vi "test_Checksum U8 - Add Protection.vi"(8 "error in (no error)":errorcluster) -> (0 "error out":errorcluster)   [LabVIEW 2019, in "Protections Unit Tests.lvclass"]
uses:
  Protections Unit Tests.lvclass
  Checksum U8/Checksum U8.lvclass
  <vilib>/addons/_JKI Toolkits/VI Tester/TestCase.llb/TestCase.lvclass
  C:/Program Files (x86)/National Instruments/LabVIEW 2019/vi.lib/addons/_JKI Toolkits/VI Tester/TestCase.llb/TestCase.lvclass
panel:
  out "Checksum U8 out":refnum<class "Checksum U8.lvclass">
  in  "Checksum U8 in":refnum<class "Checksum U8.lvclass">
  out "TestCase out":refnum<class "Protections Unit Tests.lvclass">
  in  "TestCase in":refnum<class "Protections Unit Tests.lvclass">
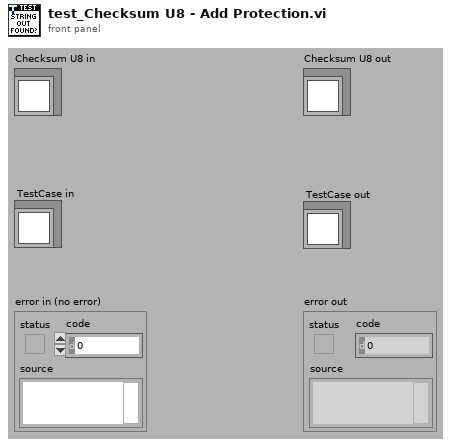
[diagram p1: front panel]
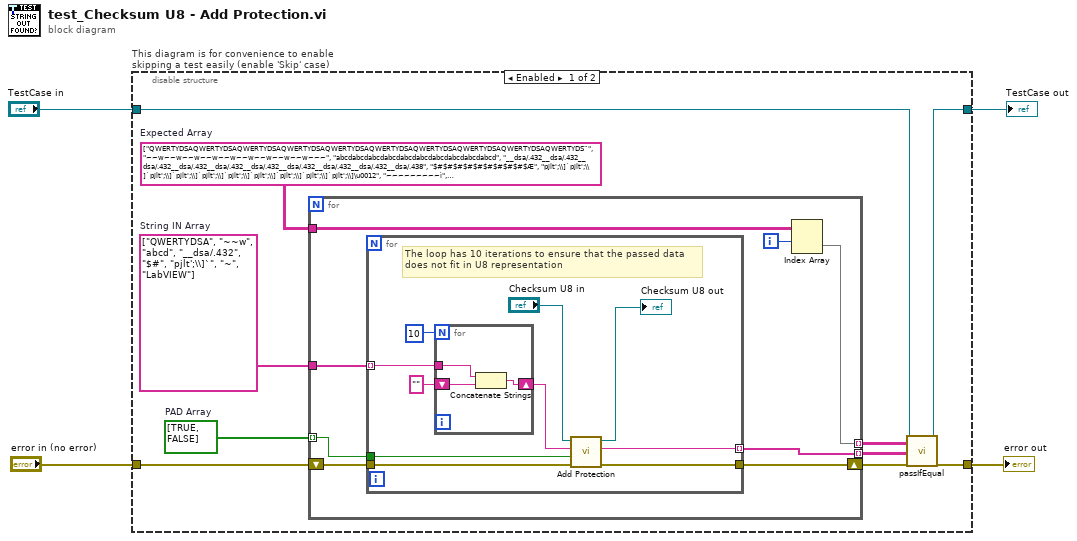
[diagram p0: block diagram]
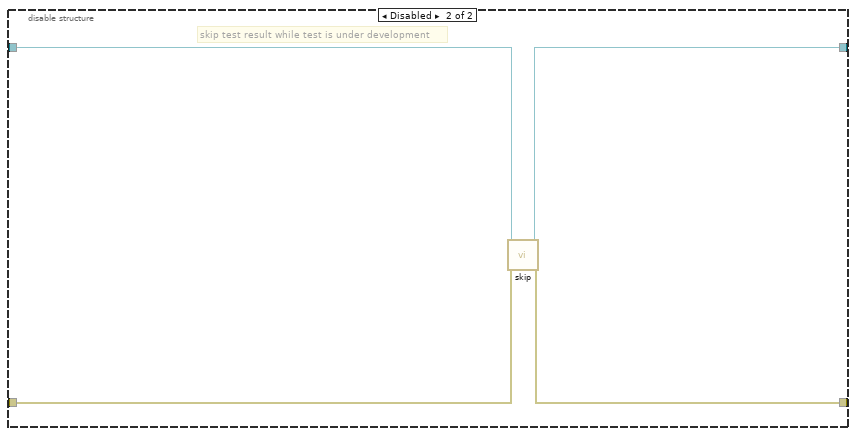
[diagram p2: hidden frame]
diagram:
  n1 = disable-structure "This diagram is for convenience to enable skipping a test easily (enable 'Skip' case)" shown="Enabled" {
    disable-tunnel: "TestCase in" -> [w12 w39]
    disable-tunnel: [w13 w37] -> w1
    disable-tunnel: [w14 w38] -> w3
    disable-tunnel: "error in (no error)" -> [w11 w36]
    frame Enabled {
      w5 = string[][] [["QWERTYDSAQWERTYDSAQWERTYDSAQWERTYDSAQWERTYDSAQWERTYDSAQWERTYDSAQWERTYDSAQWERTYDSAQWERTYDS¨", "~~w~~w~~w~~w~~w~~w~~w~~w~~w~~~", "abcdabcdabcdabcdabcdabcdabcdabcdabcdabcd", "__dsa/.432__dsa/.432__dsa/.432__dsa/.432__dsa/.432__dsa/.432__dsa/.432__dsa/.432__dsa/.432__dsa/.438", "$#$#$#$#$#$#$#$#$#$Æ", "pjlt';\\]`pjlt';\\]`pjlt';\\]`pjlt';\\]`pjlt';\\]`pjlt';\\]`pjlt';\\]`pjlt';\\]`pjlt';\\]`pjlt';\\]\u0012", "~~~~~~~~~ì", "LabVIEWLabVIEWLabVIEWLabVIEWLabVIEWLabVIEWLabVIEWLabVIEWLabVIEWLabVIEä"], ["QWERTYDSAQWERTYDSAQWERTYDSAQWERTYDSAQWERTYDSAQWERTYDSAQWERTYDSAQWERTYDSAQWERTYDSAQWERTYDSA¨", "~~w~~w~~w~~w~~w~~w~~w~~w~~w~~w~", "abcdabcdabcdabcdabcdabcdabcdabcdabcdabcdd", "__dsa/.432__dsa/.432__dsa/.432__dsa/.432__dsa/.432__dsa/.432__dsa/.432__dsa/.432__dsa/.432__dsa/.4328", "$#$#$#$#$#$#$#$#$#$#Æ", "pjlt';\\]`pjlt';\\]`pjlt';\\]`pjlt';\\]`pjlt';\\]`pjlt';\\]`pjlt';\\]`pjlt';\\]`pjlt';\\]`pjlt';\\]`\u0012", "~~~~~~~~~~ì", "LabVIEWLabVIEWLabVIEWLabVIEWLabVIEWLabVIEWLabVIEWLabVIEWLabVIEWLabVIEWä"]]  # Expected Array
      w7 = string[] ["QWERTYDSA", "~~w", "abcd", "__dsa/.432", "$#", "pjlt';\\]`", "~", "LabVIEW"]  # String IN Array
      w8 = bool[] [TRUE, FALSE]  # PAD Array
      n2 = for {
        tunnel: [w21] -> w10 mode=indexing
        shift-right: [w20] -> w9
        shift-left: w11 -> [w22]
        tunnel: w8 -> [w19] mode=indexing
        tunnel: w7 -> [w18]
        tunnel: w5 -> [w17]
        tunnel: [w16] -> w6 mode=indexing
        i -> [w15]
        n3 = for {
          tunnel: w18 -> [w30] mode=indexing
          tunnel: w22 -> [w29]
          tunnel: [w28] -> w20
          tunnel: [w27] -> w21 mode=indexing
          tunnel: w19 -> [w26]
          # "The loop has 10 iterations to ensure that the passed data\ndoes not fit in U8 representation"
          n4 = for {
            N: 10 -> [_]
            shift-right: [w35] -> w25
            shift-left: "" -> [w34]
            tunnel: w30 -> [w33]
            n5 = Concatenate Strings(w33, w34) -> (w35:string)
          }
          n6 = call-dynamic "Add Protection.vi"("error in (no error)"=w29, "Pad"=w26, "String in"=w25, "Checksum U8 in"="Checksum U8 in") -> ("error out"=w28:errorcluster, "String out"=w27:string, "Checksum U8 out"=→"Checksum U8 out":refnum<class "Checksum U8.lvclass">)  [unwired: 5 in]
        }
        n7 = Index Array "Index Array"(array=w17, index (row)=w15) -> (element=w16:string[])  [unwired: 1 in]
      }
      n8 = call-dynamic "passIfEqual.vi"("error in (no error)"=w9, "y"=w10, "x"=w6, "TestCase in"=w12) -> ("error out"=w14:errorcluster, "TestCase out"=w13:refnum<class "Protections Unit Tests.lvclass">)  [unwired: 6 in]
    }
    frame Disabled {
      # "skip test result while test is under development"
      n9 = call <vilib>:"skip.vi"("error in (no error)"=w36, "TestCase in"=w39) -> ("error out"=w38:errorcluster, "TestCase out"=w37:refnum<class "Protections Unit Tests.lvclass">)  [unwired: 8 in]
    }
  }
  "error out" <- w3
  "TestCase out" <- w1
